vi "Log Header Data Msg.vi"(8 "error in (no error)":errorcluster, 10 "read buffer":string, 11 "Queue in":refnum<queue>) -> (0 "error out":errorcluster)   [LabVIEW 2018, in "Logging.lvlib"]
uses:
  Logging.lvlib
  Support/Message Queue/Message Cluster.ctl
  Support/Message Queue/Enqueue Message (Single).vi
  support/Message Queue/Message Queue.lvlib
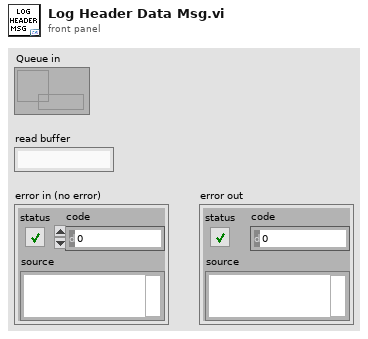
[diagram p1: front panel]
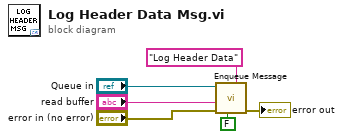
[diagram p0: block diagram]
diagram:
  n1 = call-poly "Enqueue Message.vi"("Priority Message? (F)"=FALSE, "error in (no error)"="error in (no error)", "Message Data"="read buffer", "Message"="Log Header Data", "Message Queue"="Queue in") -> ("error out"=→"error out":errorcluster)  [unwired: 5 in, 1 out]
